vi "Celsius to Fahrenheit with Kelvin.vi"() -> ()   [LabVIEW 2019]
panel:
  in  "Kelvin":dbl(slide) scale=100.0..200.0
  out "Fahrenheit":dbl(slide) scale=32.0..212.0
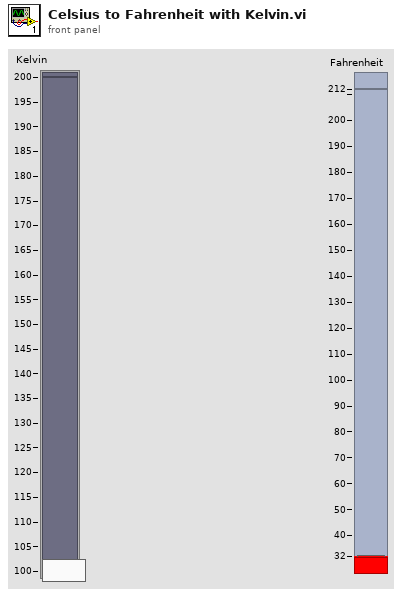
[diagram p1: front panel]
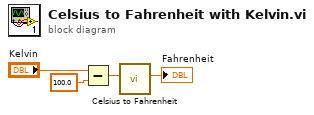
[diagram p0: block diagram]
diagram:
  n1 = Subtract(x="Kelvin", y=100.0) -> (x-y=w1:dbl)
  n2 = call "Celsius to Fahrenheit.vi"("Celsius"=w1) -> ("Fahrenheit"=→"Fahrenheit":dbl)  [unwired: 10 in]
